vi "Get Languages.vi"(8 "error in":errorcluster) -> (0 "error out":errorcluster, 2 "Languages":string[](array[string]))   [LabVIEW 2017, in "JKI Simple Localization.lvlib"]
doc: "Returns a list of all languages available in the current dictionary."
uses:
  JKI Simple Localization.lvlib
  Private/Definitions/Translation.Action.ctl
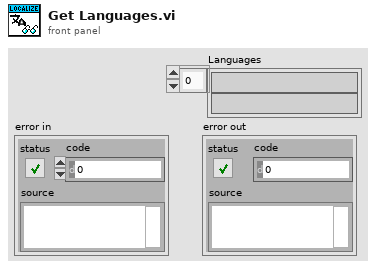
[diagram p1: front panel]
types:
  T1 = typedef "JKI Simple Localization.lvlib/Translation.Action.ctl" = enum16{"Read Dictionary", "Translate VIs", "Register VI", "Get Languages", "Translate Phrase", "Translate VI", "Unregister"}
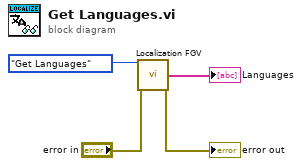
[diagram p0: block diagram]
diagram:
  n1 = call "Localization FGV.vi"("Action"=Translation.Action."Get Languages", "error in"="error in") -> ("Languages"=→"Languages":string[], "error out"=→"error out":errorcluster)  [unwired: 9 in, 3 out]
